vi "GlobalStop.vi"() -> ()   [LabVIEW 2013]
panel:
  out "stop":bool
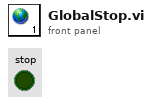
[diagram p1: front panel]
diagram:
